vi "test_libssh2_userauth_password.vi"() -> ()   [LabVIEW 2017, in "integration_tests.lvlib"]
uses:
  integration_tests.lvlib
  libssh2/libssh2_session_handshake_tcp.vi
  libssh2/libssh2_init_default.vi
  libssh2/libssh2_session_init_ex.vi
  <vilib>/Utility/tcp.llb/TCP Get Raw Net Object.vi
  libssh2/libssh2_session_handshake_socket.vi
  libssh2/libssh2_userauth_password_ex.vi
  libssh2/libssh2.lvlib
  support/support.lvlib
  <vilib>/PNR/Transparent Assertions/Transparent Assertions/Transparent Assertions.lvlib
panel:
  out "error out":errorcluster
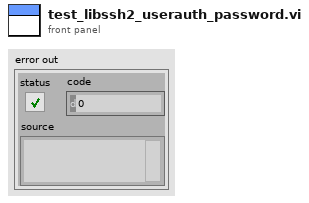
[diagram p1: front panel]
types:
  T1 = typedef "libssh2.lvlib/Session Refnum.ctl" = refnum<k1>
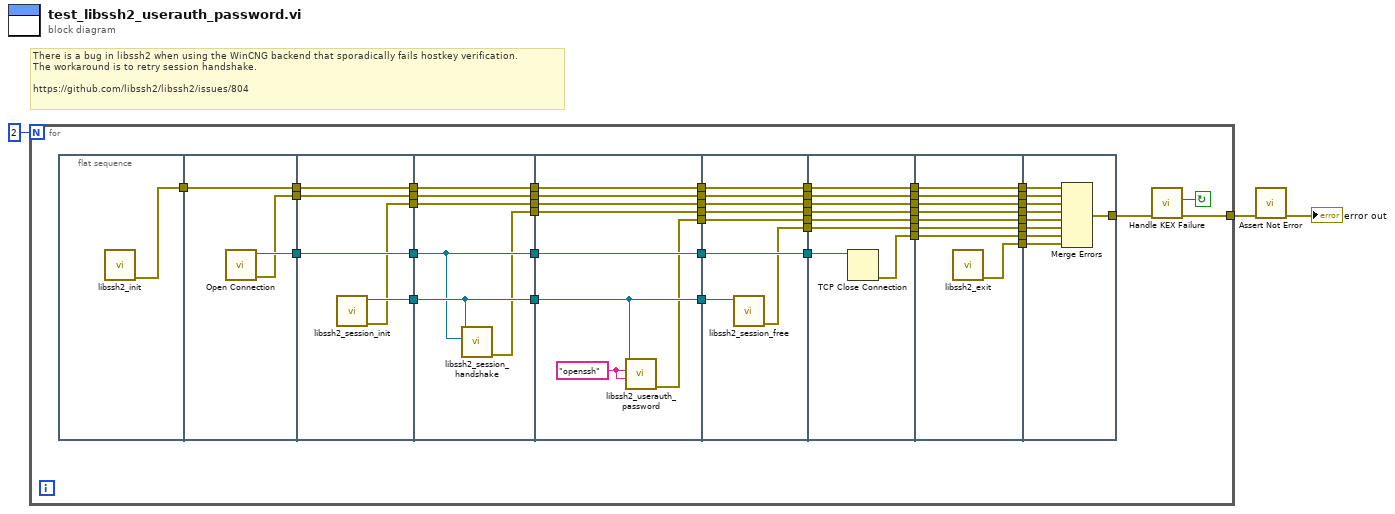
[diagram p0: block diagram]
diagram:
  # "There is a bug in libssh2 when using the WinCNG backend that sporadically fails hostkey verification.\nThe workaround is to retry session handshake.\n\nhttps://github.com/libssh2/libssh2/issues/804"
  n1 = for {
    N: 2 -> [_]
    tunnel: [w8] -> w2
    stop <- w9 continue-if-true
    n2 = flat-sequence {
      tunnel: [w51] -> w50
      tunnel: [w54] -> w49
      tunnel: w50 -> [w53]
      tunnel: [w53] -> w48
      tunnel: [w52] -> w47
      tunnel: w49 -> [w59]
      tunnel: [w59] -> w46
      tunnel: w48 -> [w58]
      tunnel: [w58] -> w45
      tunnel: w47 -> [w57]
      tunnel: [w57] -> w44
      tunnel: [w56] -> w43
      tunnel: [w55] -> w42
      tunnel: w46 -> [w61]
      tunnel: [w61] -> w41
      tunnel: w45 -> [w65]
      tunnel: [w65] -> w40
      tunnel: w44 -> [w64]
      tunnel: [w64] -> w39
      tunnel: [w63] -> w38
      tunnel: w43 -> [w63]
      tunnel: w42 -> [w62]
      tunnel: [w62] -> w37
      tunnel: [w60] -> w36
      tunnel: w41 -> [w73]
      tunnel: [w73] -> w35
      tunnel: w40 -> [w72]
      tunnel: [w72] -> w34
      tunnel: w39 -> [w71]
      tunnel: [w71] -> w33
      tunnel: w38 -> [w68]
      tunnel: w37 -> [w70]
      tunnel: [w70] -> w32
      tunnel: w36 -> [w69]
      tunnel: [w69] -> w31
      tunnel: [w68] -> w30
      tunnel: [w66] -> w7
      tunnel: w35 -> [w81]
      tunnel: [w81] -> w29
      tunnel: w34 -> [w80]
      tunnel: [w80] -> w28
      tunnel: w33 -> [w79]
      tunnel: [w79] -> w27
      tunnel: w32 -> [w78]
      tunnel: [w78] -> w26
      tunnel: w31 -> [w77]
      tunnel: [w77] -> w25
      tunnel: [w76] -> w24
      tunnel: w30 -> [w75]
      tunnel: w7 -> [w74]
      tunnel: [w74] -> w6
      tunnel: w29 -> [w89]
      tunnel: w28 -> [w88]
      tunnel: [w88] -> w23
      tunnel: w27 -> [w87]
      tunnel: [w87] -> w22
      tunnel: [w86] -> w21
      tunnel: w26 -> [w85]
      tunnel: [w85] -> w20
      tunnel: w25 -> [w84]
      tunnel: [w84] -> w19
      tunnel: [w83] -> w18
      tunnel: w24 -> [w83]
      tunnel: w6 -> [w82]
      tunnel: [w82] -> w5
      tunnel: w23 -> [w97]
      tunnel: [w97] -> w17
      tunnel: w22 -> [w96]
      tunnel: [w96] -> w16
      tunnel: w21 -> [w95]
      tunnel: [w95] -> w15
      tunnel: [w94] -> w14
      tunnel: w20 -> [w93]
      tunnel: [w93] -> w13
      tunnel: w19 -> [w92]
      tunnel: [w92] -> w12
      tunnel: [w91] -> w11
      tunnel: w18 -> [w91]
      tunnel: w5 -> [w90]
      tunnel: [w90] -> w4
      tunnel: w17 -> [w106]
      tunnel: w16 -> [w105]
      tunnel: w15 -> [w104]
      tunnel: w14 -> [w103]
      tunnel: w13 -> [w102]
      tunnel: w12 -> [w101]
      tunnel: w11 -> [w100]
      tunnel: [w99] -> w10
      tunnel: w4 -> [w98]
      frame #0 {
        n3 = call-poly "libssh2_init.vi"() -> ("error out"=w51:errorcluster)  [unwired: 11 in]
      }
      frame #1 {
        n4 = call "Open Connection.vi"() -> ("error out"=w52:errorcluster, "connection ID"=w54:refnum<k5>)  [unwired: 10 in]
      }
      frame #2 {
        n5 = call "libssh2_session_init.vi"() -> ("error out"=w55:errorcluster, "session"=w56:T1)  [unwired: 10 in]
      }
      frame #3 {
        n6 = call-poly "libssh2_session_handshake.vi"("tcp connection"=w61, "session"=w63) -> ("error out"=w60:errorcluster)  [unwired: 9 in]
      }
      frame #4 {
        w67 = "openssh" ("username")
        n7 = call "libssh2_userauth_password.vi"("password"=w67, "username"=w67, "session"=w68) -> ("error out"=w66:errorcluster)  [unwired: 8 in]
      }
      frame #5 {
        n8 = call "libssh2_session_free.vi"("session"=w75) -> ("error out"=w76:errorcluster)  [unwired: 10 in]
      }
      frame #6 {
        n9 = TCP Close Connection(connection ID=w89) -> (error out=w86:errorcluster)  [unwired: 2 in, 1 out]
      }
      frame #7 {
        n10 = call "libssh2_exit.vi"() -> ("error out"=w94:errorcluster)  [unwired: 11 in]
      }
      frame #8 {
        n11 = Merge Errors(w106, w105, w102, w101, w98, w100, w104, w103) -> (w99:errorcluster)
      }
    }
    n12 = call "Handle KEX Failure.vi"("error in (no error)"=w10) -> ("error out"=w8:errorcluster, "KEX Failure"=w9:bool)  [unwired: 9 in]
  }
  n13 = call <vilib>:"Assert Not Error.vi"("error in (no error)"=w2) -> ("error out"=→"error out":errorcluster)  [unwired: 10 in]
